vi "Set MICS Channel.vi"(2 "MICS_Channel":dbl) -> (0 "error out":errorcluster)   [LabVIEW 2010]
uses:
  MICS_Channel Global.vi
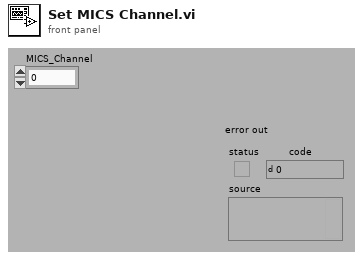
[diagram p1: front panel]
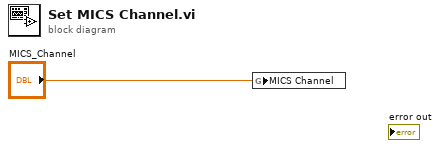
[diagram p0: block diagram]
diagram:
  n1 = global write "MICS_Channel Global.vi" "MICS Channel"("MICS_Channel") -> ()
